vi "Read Deg.vi"(8 "error out":errorcluster, 11 "VISA resource name out":refnum<visa-resource-name>) -> (0 "error out 2":errorcluster caption="error out", 2 "角度":dbl, 3 "VISA resource name out 2":refnum<visa-resource-name>)   [LabVIEW 2015]
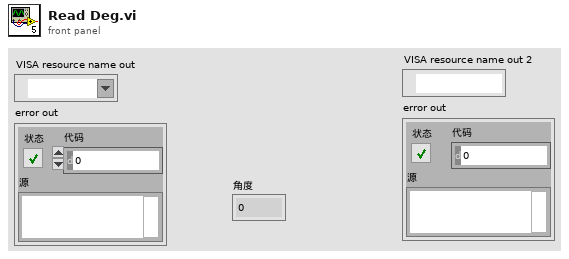
[diagram p1: front panel]
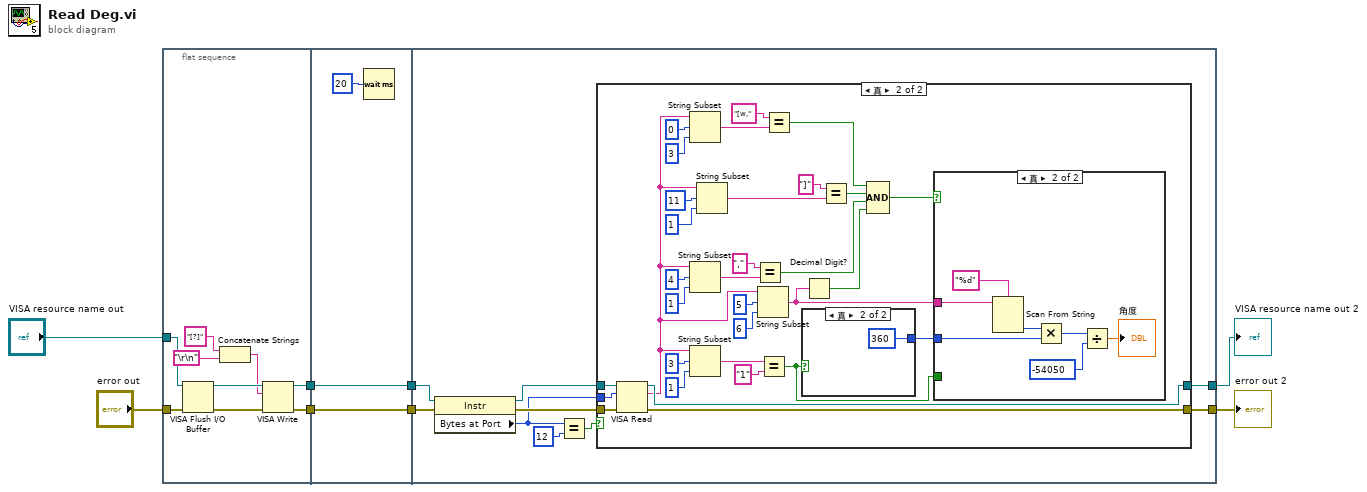
[diagram p0: block diagram]
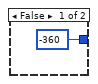
[diagram p3: hidden frame]
diagram:
  n1 = flat-sequence {
    tunnel: "VISA resource name out" -> [w12]
    tunnel: "error out" -> [w11]
    tunnel: [w10] -> w8
    tunnel: [w9] -> w7
    tunnel: [w19] -> w6
    tunnel: w8 -> [w19]
    tunnel: [w18] -> w5
    tunnel: w7 -> [w18]
    tunnel: w6 -> [w29]
    tunnel: w5 -> [w28]
    tunnel: [w22] -> w2
    tunnel: [w21] -> w1
    frame #0 {
      n2 = VISA Flush I/O Buffer(VISA resource name=w12, error in (no error)=w11) -> (VISA resource name out=w16:refnum<visa-resource-name>, error out=w17:errorcluster)  [unwired: 1 in]
      n3 = Concatenate Strings("[?]" ("字符串"), "\r\n") -> (w13:string)
      n4 = VISA Write(VISA resource name=w16, write buffer=w13, error in (no error)=w17) -> (VISA resource name out=w10:refnum<visa-resource-name>, error out=w9:errorcluster)  [unwired: 1 out]
    }
    frame #1 {
      n5 = Wait (ms)(milliseconds to wait=u32 20 ("等待时间（毫秒）")) -> ()  [unwired: 1 out]
    }
    frame #2 {
      n6 = property class="Instr"(reference=w29, error in=w28) -> (reference out=w24:refnum<visa-resource-name>, error out=w25:errorcluster, "Bytes at Port"=w23:u32)
      n7 = Equal?(x=w23, y=u32 12) -> (x = y?=w26:bool)
      n8 = case shown="真" w26 {
        tunnel: w25 -> [w30 w63]
        tunnel: w24 -> [w31 w62]
        tunnel: w23 -> [_ w61]
        tunnel: [w31 w41] -> w22
        tunnel: [w30 w40] -> w21
        frame False {
        }
        frame True {
          n9 = VISA Read(VISA resource name=w62, byte count=w61, error in (no error)=w63) -> (VISA resource name out=w41:refnum<visa-resource-name>, read buffer=w38:string, error out=w40:errorcluster)  [unwired: 1 out]
          n10 = String Subset(string=w38, offset (0)=0 ("偏移量(0)"), length (rest)=3 ("长度（剩余）")) -> (substring=w51:string)
          n11 = String Subset(string=w38, offset (0)=4 ("偏移量(0)"), length (rest)=1 ("长度（剩余）")) -> (substring=w55:string)
          n12 = String Subset(string=w38, offset (0)=3 ("偏移量(0)"), length (rest)=1 ("长度（剩余）")) -> (substring=w33:string)
          n13 = String Subset(string=w38, offset (0)=11 ("偏移量(0)"), length (rest)=1 ("长度（剩余）")) -> (substring=w53:string)
          n14 = Equal?(x=",", y=w55) -> (x = y?=w59:bool)
          n15 = String Subset(string=w38, offset (0)=5 ("偏移量(0)"), length (rest)=6 ("长度（剩余）")) -> (substring=w39:string)
          n16 = Equal?(x=w33, y="1") -> (x = y?=w32:bool)
          n17 = Equal?(x="[w,", y=w51) -> (x = y?=w57:bool)
          n18 = case shown="真" w32 {
            tunnel: [-360 ("y") 360 ("y")] -> w34
            frame False {
            }
            frame True {
            }
          }
          n19 = Decimal Digit?(1:w39) -> (0:w60:bool)
          n20 = Equal?(x="]", y=w53) -> (x = y?=w58:bool)
          n21 = Compound Arithmetic op=AND(w57, w58, w59, w60) -> (w42:bool)
          n22 = case shown="真" w42 {
            tunnel: w39 -> [_ w69]
            tunnel: w34 -> [_ w67]
            tunnel: w32 -> [_ _]
            frame False {
            }
            frame True {
              n23 = Scan From String(format string="%d" ("格式字符串"), input string=w69) -> (output 1=w68:i32)  [unwired: 3 in, 3 out]
              n24 = Multiply(x=w68, y=w67) -> (x*y=w72:i32)
              n25 = Divide(x=w72, y=-54050) -> (x/y=→"角度":dbl)
            }
          }
        }
      }
    }
  }
  "VISA resource name out 2" <- w2
  "error out 2" <- w1
